vi "OpenAcquisitionFileForWrite-subvi.vi"(8 "Number of acquisition files":i32, 9 "Existing directory to over-write":path, 10 "Use new?":bool, 11 "New directory to create":path) -> (0 "OK?":bool, 3 "Sequence files handle":T1)   [LabVIEW 2014]
uses:
  Camera & acquisition VIs/Globals/Initilize Globals.vi
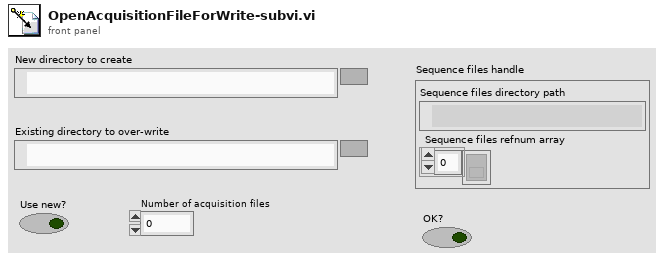
[diagram p1: front panel]
types:
  T1 = cluster{"Sequence files directory path":path, "Sequence files refnum array":refnum<file>[]}
  T2 = enum16{"open", "replace", "create", "open or create", "replace or create", "replace or create with confirmation"}
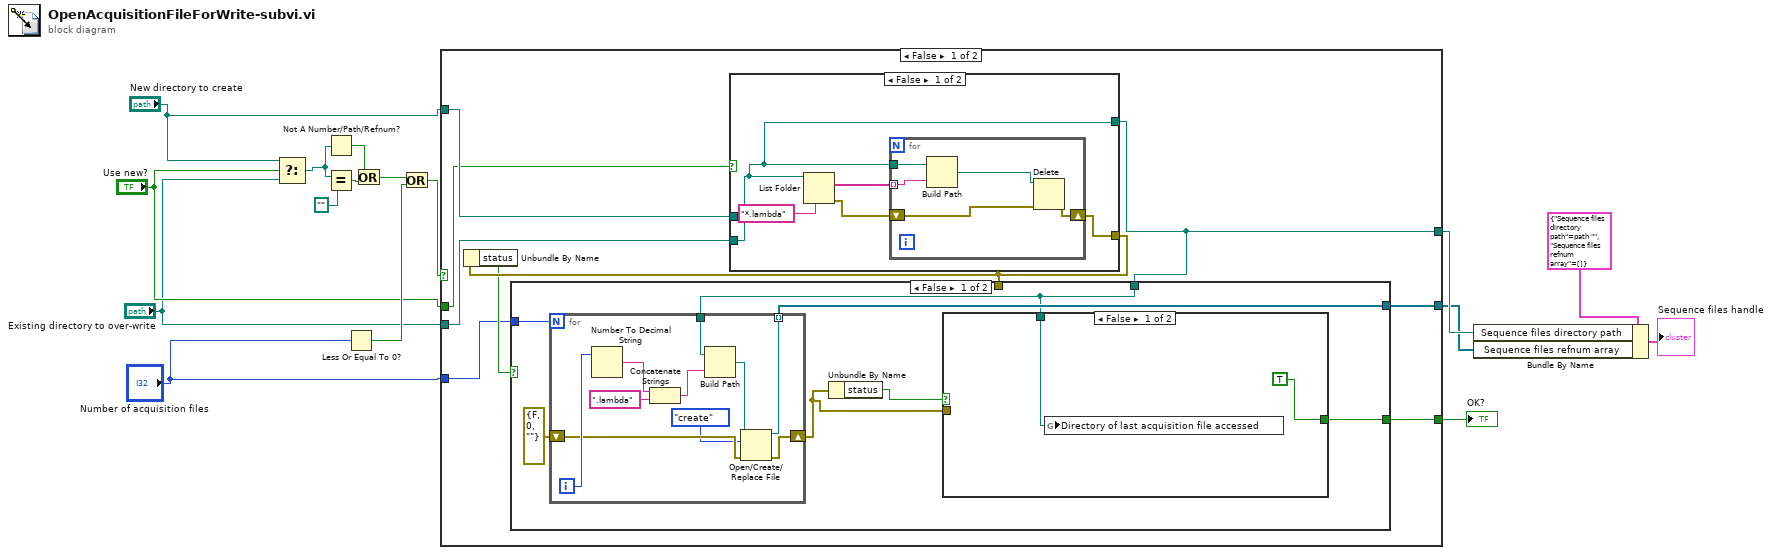
[diagram p0: block diagram]
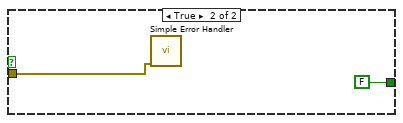
[diagram p2: hidden frame]
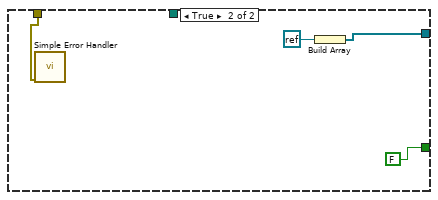
[diagram p3: hidden frame]
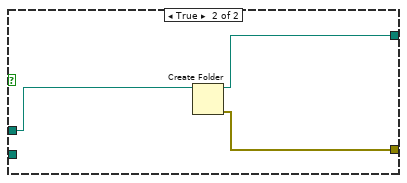
[diagram p4: hidden frame]
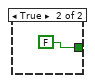
[diagram p5: hidden frame]
diagram:
  n1 = Select(t="New directory to create", s="Use new?", f="Existing directory to over-write") -> (s? t:f=w14:path)
  n2 = Not A Number/Path/Refnum?(number/path/refnum=w14) -> (NaN/Path/Refnum?=w15:bool)
  n3 = Equal?(x=w14, y=path "") -> (x = y?=w16:bool)
  n4 = Less Or Equal To 0?(x="Number of acquisition files") -> (x <= 0?=w11:bool)
  n5 = Or(x=w15, y=w16) -> (x .or. y?=w12:bool)
  n6 = Or(x=w12, y=w11) -> (x .or. y?=w10:bool)
  n7 = case shown="False" w10 {
    tunnel: "New directory to create" -> [w25 _]
    tunnel: "Use new?" -> [w18 _]
    tunnel: "Number of acquisition files" -> [w17 _]
    tunnel: "Existing directory to over-write" -> [w24 _]
    tunnel: [w21 _] -> w3
    tunnel: [w20 _] -> w2
    tunnel: [w19 FALSE] -> w1
    frame False {
      n8 = case shown="False" w18 {
        tunnel: w25 -> [_ w63]
        tunnel: w24 -> [w53 _]
        tunnel: [w53 w62] -> w21
        tunnel: [w52 w61] -> w23
        frame False {
          n9 = List Folder(path=w53, pattern="*.lambda") -> (filenames=w55:string[], error out=w54:errorcluster)  [unwired: 1 in, 3 out]
          n10 = for {
            tunnel: w55 -> [w56] mode=indexing
            shift-right: [w58] -> w52
            shift-left: w54 -> [w59]
            tunnel: w53 -> [w57]
            n11 = Build Path(base path=w57, name or relative path=w56) -> (appended path=w60:path)
            n12 = Delete(path (use dialog)=w60, error in=w59) -> (error out=w58:errorcluster)  [unwired: 5 out]
          }
        }
        frame True {
          n13 = Create Folder(path (use dialog)=w63) -> (created path=w62:path, error out=w61:errorcluster)  [unwired: 1 in, 2 out]
        }
      }
      n14 = Unbundle By Name(w23) -> ("status"=w22:bool)
      n15 = case shown="False" w22 {
        tunnel: w23 -> [_ w50]
        tunnel: w21 -> [w29 _]
        tunnel: [w30 w47] -> w20
        tunnel: [w28 FALSE] -> w19
        tunnel: w17 -> [w26 _]
        frame False {
          n16 = for {
            N: w26 -> [_]
            shift-right: [w42] -> w27
            shift-left: errorcluster {"status"=FALSE, "code"=0, "source"=""} ("Error In") -> [w43]
            tunnel: w29 -> [w40]
            tunnel: [w38] -> w30 mode=indexing
            i -> [w46]
            n17 = Number To Decimal String(number=w46) -> (decimal integer string=w45:string)  [unwired: 1 out]
            n18 = Concatenate Strings(w45, ".lambda" ("string")) -> (w44:string)
            n19 = Build Path(base path=w40, name or relative path=w44) -> (appended path=w39:path)
            n20 = Open/Create/Replace File(file path (use dialog)=w39, error in=w43, operation (0:open)=T2."create") -> (refnum out=w38:refnum<file>, error out=w42:errorcluster)  [unwired: 4 out]
          }
          n21 = Unbundle By Name(w27) -> ("status"=w31:bool)
          n22 = case shown="False" w31 {
            tunnel: w29 -> [w34 _]
            tunnel: [TRUE FALSE] -> w28
            tunnel: w27 -> [_ w35]
            frame False {
              n23 = global write "Initilize Globals.vi" "Directory of last acquisition file accessed"(w34) -> ()
            }
            frame True {
              n24 = call <vilib>:"Simple Error Handler.vi"("error in (no error)"=w35) -> ()  [unwired: 4 in, 5 out]
            }
          }
        }
        frame True {
          n25 = call <vilib>:"Simple Error Handler.vi"("error in (no error)"=w50) -> ()  [unwired: 4 in, 5 out]
          n26 = Build Array(refnum<k0> refnum) -> (w47:refnum<k0>[])
        }
      }
    }
    frame True {
    }
  }
  "OK?" <- w1
  n27 = Bundle By Name(cluster=T1 {"Sequence files directory path"=path "", "Sequence files refnum array"=[]} ("Sequence files handle"), "Sequence files directory path"=w3, "Sequence files refnum array"=w2) -> (→"Sequence files handle":T1)
